vi "Stub_Custom Error.vi"() -> (3 "error out":errorcluster)   [LabVIEW 2019]
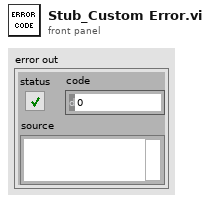
[diagram p1: front panel]
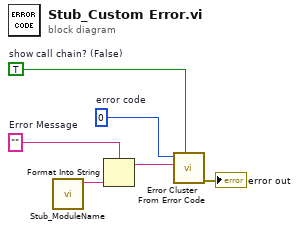
[diagram p0: block diagram]
diagram:
  w4 = 0  # error code
  w1 = ""  # Error Message
  w5 = TRUE  # show call chain? (False)
  n1 = call "Stub_ModuleName.vi"() -> ("Module Name"=w3:string)  [unwired: 11 in]
  n2 = Format Into String(format string=w1, w3) -> (resulting string=w2:string)  [unwired: 2 in, 1 out]
  n3 = call <vilib>:"Error Cluster From Error Code.vi"("show call chain? (False)"=w5, "error message (\"\")"=w2, "error code (0)"=w4) -> ("error out"=→"error out":errorcluster)  [unwired: 6 in]
